vi "ZipPlugins.vi"(8 "error in (no error)":errorcluster, 11 "Workspace path":path) -> (0 "error out":errorcluster)   [LabVIEW 2017]
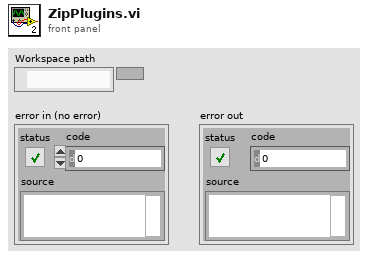
[diagram p1: front panel]
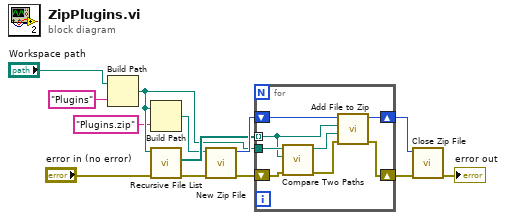
[diagram p0: block diagram]
diagram:
  n1 = Build Path(base path="Workspace path", name or relative path="Plugins") -> (appended path=w8:path)
  n2 = Build Path(base path=w8, name or relative path="Plugins.zip") -> (appended path=w6:path)
  n3 = call <vilib>:"Recursive File List.vi"("error in (no error)"="error in (no error)", "Folder Path"=w8) -> ("error out"=w4:errorcluster, "All Files in Dir"=w9:path[])  [unwired: 5 in, 3 out]
  n4 = call <vilib>:"New Zip File.vi"("error in (no error)"=w4, "target"=w6) -> ("error out"=w7:errorcluster, "zip file out"=w10:i64)  [unwired: 3 in, 1 out]
  n5 = for {
    tunnel: w8 -> [w19]
    tunnel: w9 -> [w17] mode=indexing
    shift-right: [w15] -> w11
    shift-left: w7 -> [w21]
    shift-right: [w14] -> w12
    shift-left: w10 -> [w16]
    n6 = call <vilib>:"Compare Two Paths.vi"("error in (no error)"=w21, "Path 2"=w17, "Path 1"=w19) -> ("error out"=w20:errorcluster, "Relative Path from 1 to 2"=w18:path)  [unwired: 5 in, 2 out]
    n7 = call <vilib>:"Add File to Zip.vi"("error in (no error)"=w20, "destination path in zip"=w18, "source file path"=w17, "zip file in"=w16) -> ("error out"=w15:errorcluster, "zip file out"=w14:i64)  [unwired: 6 in]
  }
  n8 = call <vilib>:"Close Zip File.vi"("error in (no error)"=w11, "zip file in"=w12) -> ("error out"=→"error out":errorcluster)  [unwired: 1 in, 4 out]
